vi "Position Peek Window.vi"(8 "Error In":errorcluster, 9 "Subpanel":refnum<vi>, 10 "Active Components":T1, 11 "PeekVI Reference":refnum<vi>) -> (0 "error out":errorcluster)   [LabVIEW 2020, in "Peek Window.lvlib"]
uses:
  Peek Window.lvlib
  Open Diagram Argument--cluster.ctl
  <vilib>/Utility/miscctls.llb/LVPointTypeDef.ctl
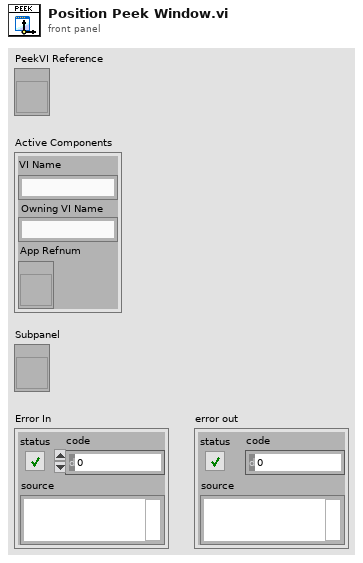
[diagram p1: front panel]
types:
  T1 = typedef "Peek Window.lvlib/Open Diagram Argument--cluster.ctl" = cluster{"VI Name":string, "Owning VI Name":string, "App Refnum":refnum<vi>}
  T2 = typedef "LVPointTypeDef.ctl" = cluster{"Horizontal":i16, "Vertical":i16}
  T3 = enum32{"Invalid", "Standard", "Closed", "Hidden", "Minimized", "Maximized"}
  T4 = typedef "LVRectTypeDef.ctl" = cluster{"Left":i16, "Top":i16, "Right":i16, "Bottom":i16}
  T5 = cluster{"Bounds":cluster{"Left":i16, "Top":i16, "Right":i16, "Bottom":i16}, "Depth":i16}
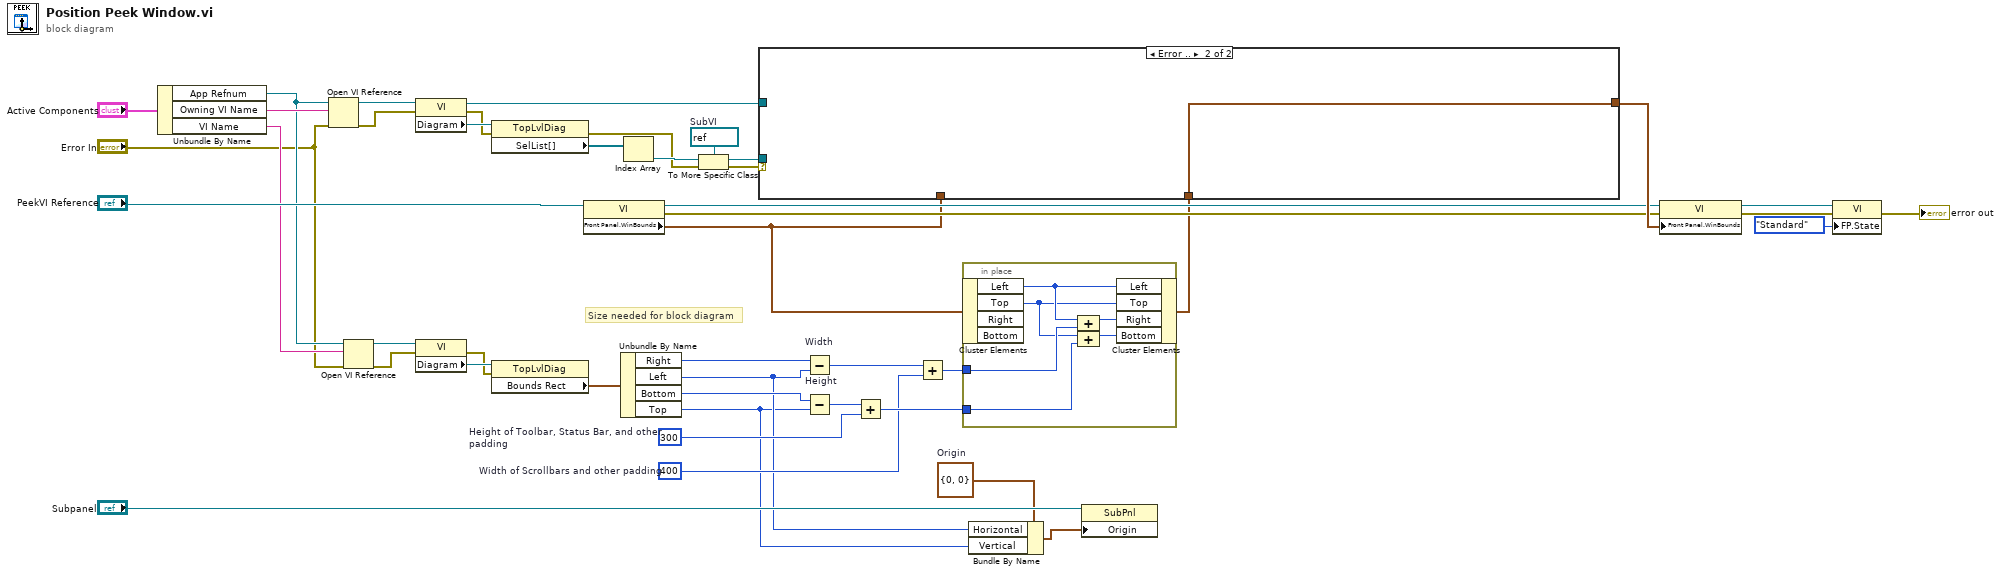
[diagram p0: block diagram]
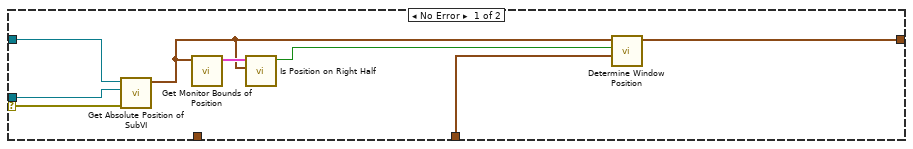
[diagram p2: hidden frame]
diagram:
  w5 = T2 {"Horizontal"=0, "Vertical"=0}  # Origin
  w7 = i16 400  # Width of Scrollbars and other padding
  w10 = i16 300  # Height of Toolbar, Status Bar, and other padding
  w30 = refnum<vi> refnum  # SubVI
  # "Size needed for block diagram"
  n1 = Unbundle By Name("Active Components") -> ("App Refnum"=w22:refnum<vi>, "Owning VI Name"=w38:string, "VI Name"=w23:string)
  n2 = Open VI Reference(application reference (local)=w22, vi path=w38, error in (no error)="Error In") -> (vi reference=w37:refnum<vi>, error out=w36:errorcluster)  [unwired: 3 in]
  n3 = Open VI Reference(application reference (local)=w22, vi path=w23, error in (no error)="Error In") -> (vi reference=w20:refnum<vi>, error out=w19:errorcluster)  [unwired: 3 in]
  n4 = property class="VI"(reference=w37, error in=w36) -> (reference out=w28:refnum<vi>, error out=w31:errorcluster, "Diagram"=w35:refnum<vi>)
  n5 = property class="VI"(reference=w20, error in=w19) -> (error out=w17:errorcluster, "Diagram"=w18:refnum<vi>)  [unwired: 1 out]
  n6 = property class="TopLvlDiag"(reference=w35, error in=w31) -> (error out=w32:errorcluster, "SelList[]"=w34:refnum<vi>[])  [unwired: 1 out]
  n7 = property class="TopLvlDiag"(reference=w18, error in=w17) -> ("Bounds Rect"=w16:T4)  [unwired: 2 out]
  n8 = property class="VI"(reference="PeekVI Reference") -> (reference out=w41:refnum<vi>, error out=w40:errorcluster, "Front Panel.WinBounds"=w1:T4)  [unwired: 1 in]
  n9 = Unbundle By Name(w16) -> ("Right"=w14:i16, "Left"=w4:i16, "Bottom"=w13:i16, "Top"=w3:i16)
  n10 = Index Array(array=w34) -> (element=w33:refnum<vi>)  [unwired: 1 in]
  n11 = To More Specific Class(target class=w30, reference=w33, error in=w32) -> (specific class reference=w29:refnum<vi>, error out=w27:errorcluster)
  n12 = Subtract "Width"(x=w14, y=w4) -> (x-y=w12:i16)
  n13 = Subtract "Height"(x=w13, y=w3) -> (x-y=w11:i16)
  n14 = Add(x=w11, y=w10) -> (x+y=w9:i16)
  n15 = Add(x=w12, y=w7) -> (x+y=w8:i16)
  n16 = in-place {
    in-place-border: w8 -> [w48]
    in-place-border: w9 -> [w47]
    n17 = in-place-cluster #1(w1) -> ("Left"=w46:i16, "Top"=w45:i16)  [unwired: 2 out]
    n18 = Compound Arithmetic op=ADD(w46, w48) -> (w50:i16)
    n19 = Compound Arithmetic op=ADD(w45, w47) -> (w49:i16)
    n20 = in-place-cluster #1("Left"=w46, "Top"=w45, "Right"=w50, "Bottom"=w49) -> (w15:T4)
  }
  n21 = case shown="Error .." w27 {
    selector: w27 -> [w54 _]
    tunnel: [w58 w59] -> w42
    tunnel: w29 -> [w56 _]
    tunnel: w28 -> [w55 _]
    tunnel: w15 -> [w51 w59]
    tunnel: w1 -> [_ _]
    frame No Error {
      n22 = call "Get Absolute Position of SubVI.vi"("Error In"=w54, "SubVI Reference"=w56, "VI Reference"=w55) -> ("Position"=w52:cluster{i32, i32})  [unwired: 7 in, 1 out]
      n23 = call "Get Monitor Bounds of Position.vi"("Position"=w52) -> ("Monitor Bounds"=w57:T5)  [unwired: 10 in]
      n24 = call "Is Position on Right Half.vi"("Position"=w52, "Monitor Bounds"=w57) -> ("On Right?"=w53:bool)  [unwired: 9 in]
      n25 = call "Determine Window Position.vi"("Window Bounds"=w51, "On Right?"=w53, "Position"=w52) -> ("Window Bounds"=w58:T4)  [unwired: 8 in]
    }
    frame Error {
    }
  }
  n26 = Bundle By Name(cluster=w5, "Horizontal"=w4, "Vertical"=w3) -> (w2:T2)
  n27 = property class="SubPnl"(reference="Subpanel", "Origin"=w2) -> ()  [unwired: 1 in, 2 out]
  n28 = property class="VI"(reference=w41, error in=w40, "Front Panel.WinBounds"=w42) -> (reference out=w25:refnum<vi>, error out=w43:errorcluster)
  n29 = property class="VI"(reference=w25, error in=w43, "FP.State"=T3."Standard" ("Front Panel Window:State")) -> (error out=→"error out":errorcluster)  [unwired: 1 out]
